vi "Increment.vi"(10 "Index":i32, 11 "Variables in":refnum<class "Variables.lvclass">) -> (2 "Incremented":dbl, 3 "Variables out":refnum<class "Variables.lvclass">, 5 "Original":dbl)   [LabVIEW 2020, in "VolatusSeq.lvlib" / "Variables.lvclass"]
uses:
  Variables.lvclass
  Variables.lvclass/Variables.ctl
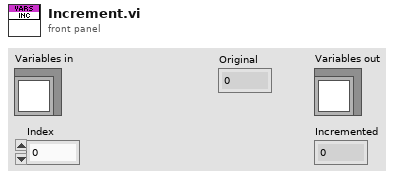
[diagram p1: front panel]
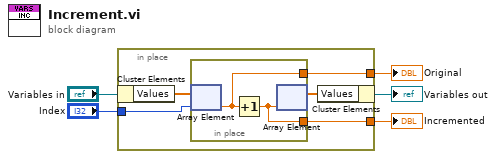
[diagram p0: block diagram]
diagram:
  n1 = in-place {
    in-place-border: "Index" -> [w9]
    in-place-border: [w7] -> w2
    in-place-border: [w6] -> w1
    n2 = in-place-cluster #1("Variables in") -> ("Values"=w10:dbl[])
    n3 = in-place {
      in-place-border: [w12] -> w7
      in-place-border: [w11] -> w6
      n4 = in-place-array #2(w10, w9) -> (w12:dbl)
      n5 = Increment(x=w12) -> (x+1=w11:dbl)
      n6 = in-place-array #2(w11) -> (w8:dbl[])  [unwired: 1 out]
    }
    n7 = in-place-cluster #1("Values"=w8) -> (→"Variables out":refnum<class "Variables.lvclass">)
  }
  "Original" <- w2
  "Incremented" <- w1
